vi "DatatoGraphNHRDC.vi"(0 "NHRDC":refnum<vi>, 1 "PlotYAxis":u32[](array[numeric]), 5 "Array":T1[](array[typedef]), 11 "error in (no error)":errorcluster) -> (4 "NHRDC":waveform(sgl)[](graph) caption="NHRRGS", 6 "Incorrect DataType?":bool, 15 "error out":errorcluster)   [LabVIEW 2018, in "AcPwrModule.lvlib"]
uses:
  AcPwrModule.lvlib
  AcPwrPlugins/NHRDCPower/TypeDefs/MeasurementData.ctl
  AcPwrPlugins/NHRDCPower/NHRDCPower.lvclass
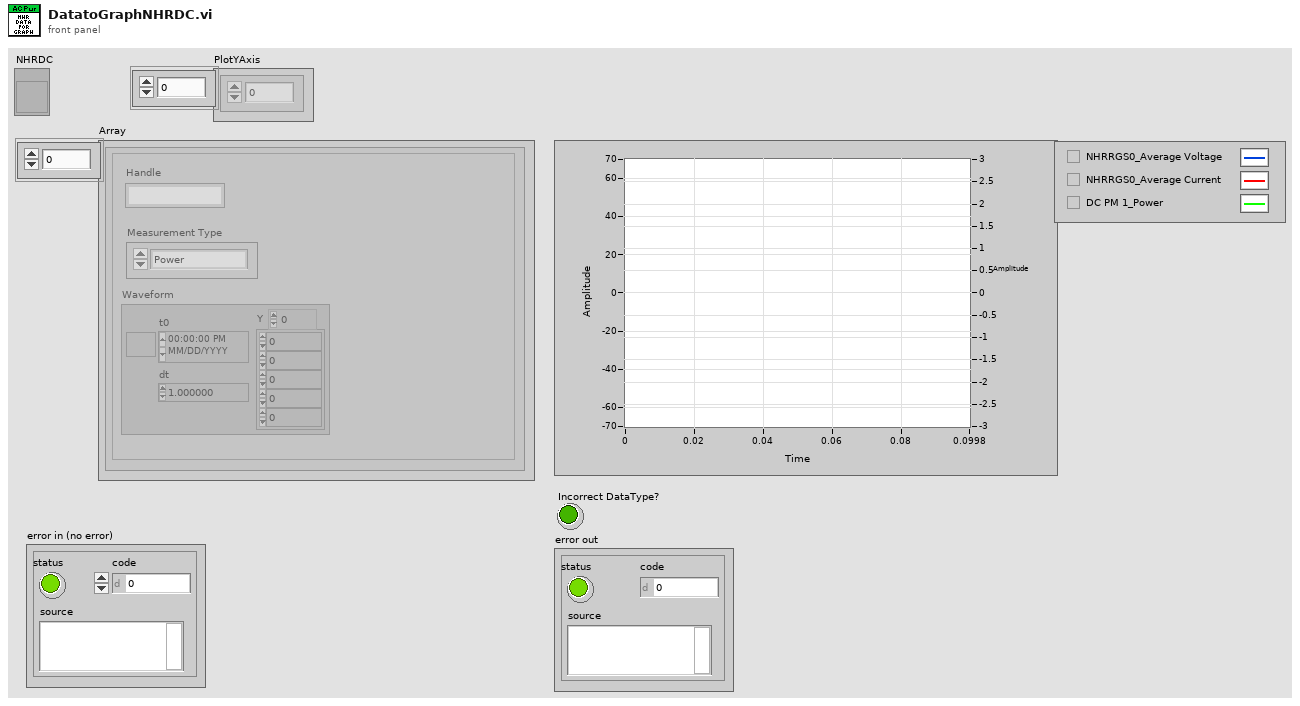
[diagram p1: front panel]
types:
  T1 = typedef "AcPwrPlugins.lvlib/NHRDCPower.lvclass/MeasurementData.ctl" = cluster{"Handle":string, "Measurement Type":enum16{"Power", "Current", "Voltage"}, "Waveform":waveform(sgl)}
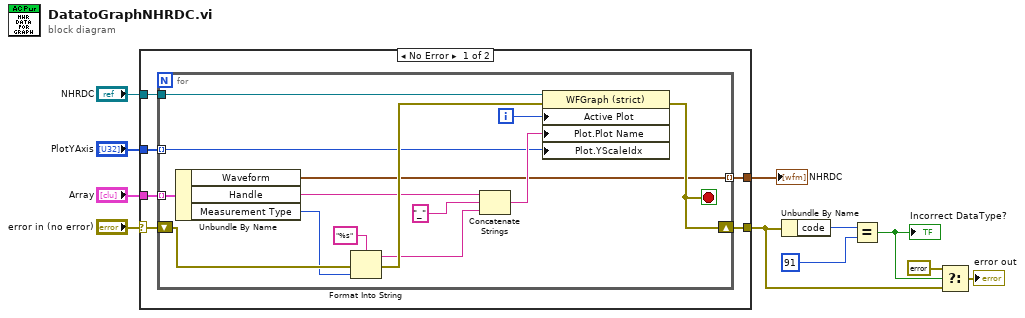
[diagram p0: block diagram]
diagram:
  n1 = case shown="No Error" "error in (no error)" {
    selector: "error in (no error)" -> [w12 w32]
    tunnel: [w17 _] -> w2
    tunnel: "Array" -> [w16 _]
    tunnel: [w15 w32] -> w4
    tunnel: "NHRDC" -> [w14 _]
    tunnel: "PlotYAxis" -> [w13 _]
    frame No Error {
      n2 = for {
        shift-right: [w21] -> w15
        shift-left: w12 -> [w24]
        tunnel: w16 -> [w31] mode=indexing
        tunnel: [w20] -> w17 mode=indexing
        tunnel: w14 -> [w23]
        tunnel: w13 -> [w22] mode=indexing
        i -> [w30]
        stop <- w21 stop-if-true
        n3 = Unbundle By Name(w31) -> ("Waveform"=w20:waveform(sgl), "Handle"=w19:string, "Measurement Type"=w18:enum16{"Power", "Current", "Voltage"})
        n4 = Format Into String(format string="%s", error in=w24, w18) -> (resulting string=w27:string, error out=w28:errorcluster)  [unwired: 1 in]
        n5 = Concatenate Strings(w19, "_" ("string"), w27) -> (w26:string)
        n6 = property on="Property Node" class="WFGraph (strict)"(reference=w23, error in=w28, "Active Plot"=w30, "Plot.Plot Name"=w26, "Plot.YScaleIdx"=w22) -> (error out=w21:errorcluster)  [unwired: 1 out]
      }
    }
    frame Error {
    }
  }
  "NHRDC" <- w2
  n7 = Unbundle By Name(w4) -> ("code"=w9:i32)
  n8 = Equal?(x=w9, y=91) -> (x = y?=w5:bool)
  "Incorrect DataType?" <- w5
  n9 = Select(t=errorcluster {"status"=FALSE, "code"=0, "source"=""} ("error IO"), s=w5, f=w4) -> (s? t:f=→"error out":errorcluster)
